vi "main.vi"() -> ()   [LabVIEW 2020]
uses:
  <vilib>/Math Plots/3D Math Plots/3D Scatter/3D Scatter XCtrl/3D Scatter.xctl
  <vilib>/Utility/miscctls.llb/LVRectTypeDef.ctl
  4961857f-4cb1-4452-8877-0132d1278599.vi
  3aed9957-f963-49bf-9f60-3d26462443e8.vi
  8fbe439c-06e5-460e-a560-e938ce784f44.vi
  460a15f0-0b3a-4794-87ef-3f3f720a4f09.vi
  13309ec4-5ddb-4caa-9ccb-149c6c5ba2b7.vi
  adf563d6-8bae-41a4-be26-81c21254c55c.vi
  <vilib>/Utility/inputDevices.llb/keyboardAcquire.vi
  <vilib>/Math Plots/3D Math Plots/3D Scatter/3D Scatter Datatype/Public/Plot Helper (Vector).vi
  <vilib>/Utility/inputDevices.llb/closeKeyboard.vi
  <vilib>/Math Plots/3D Math Plots/3D Scatter/3D Scatter Datatype/3D Scatter Datatype.lvclass
panel:
  in  "Motion Tab":enum32{"POSITION", "MEASUREMENT"}(tab)
  in  "Run Program":bool
  in  "Select Program":string(combo)="NONE"
  out "1st Key":T1(ring)
  in  "Next Button":bool
  in  "Previous Button":bool
  in  "Up Button":bool
  in  "Down Button":bool
  in  "Jog Axes":bool
  in  "Menu Ring":string(combo)
  in  "Move":bool
  in  "Axis 1 Distance":dbl format="%.2g"
  in  "Axis 0 Distance":dbl format="%.2g"
  in  "Axis 0 Speed":dbl format="%.2g"
  in  "Axis 1 Speed":dbl format="%.2g"
  in  "Axis 1 Acc":dbl format="%.2g"
  in  "Axis 0 Acc":dbl format="%.2g"
  in  "Set Parameters 2":bool
  in  "Axis 1 Jogspeed":dbl format="%.2g"
  in  "Axis 0 Jogspeed":dbl format="%.2g"
  in  "Track Offset\n(deg)":dbl format="%.2g"
  out "Data Points Logged":i32
  out "Laser Logging?":bool
  in  "Measurement\nAxis":i32(ring) items=["X Axis", "Y Axis"]
  in  "Travel Speed\n(mm/s)":dbl format="%.2g"
  in  "Set Parameters":bool
  in  "Ramp Distance\n(mm)":dbl min=0.0 format="%.2g"
  in  "Num Tracks":i32
  in  "Evaluation Length\n(mm)":dbl min=-90.0 max=90.0 format="%.2g"
  in  "Test Name":string
  out "Travel Dist":dbl
  in  "Travel Acc\n(mm/s2)":dbl format="%.2g"
  in  "Start Measurement":bool
  in  "Save Directory":path
  in  "STOP":bool
  in  "Setup Tab":enum32{"SETUP", "MONITORING", "ERRORS"}(tab)
  in  "Laser Offset":dbl
  in  "Home Axis":bool
  in  "Plot Laser Data":bool
  out "IsOpen":bool
  in  "Connection?":refnum<k7>(container)
  in  "Connect  to Controller":bool=TRUE
  in  "Set Parameters":bool
  in  "Controller Connection Type":string(combo)="2"
  out "Controller Type":string
  out "Product Name":string
  out "Version":string
  out "Serial Port":fxp<+,3,3>
  in  "Axis Enable":bool
  out "Lin Enc Pos":dbl format="%.3g"
  out "A Error":bool
  out "X Error":bool
  out "Axis 0 Position":dbl format="%.3f"
  out "Axis 0 End Pos":dbl format="%.3g"
  out "Axis 0 Velocity":dbl format="%.3g"
  out "A0 Remaining":dbl format="%.3g"
  out "XY Graph":cluster{"X":dbl, "Y":dbl}[](graph)
  out "A1 Remaining":dbl format="%.3g"
  out "Axis 1 End Pos":dbl format="%.3g"
  out "Axis 1 Velocity":dbl format="%.3g"
  out "Axis 1 Position":dbl format="%.3g"
  out "Rot Enc Pos":dbl format="%.3g"
  out "Loop Time (us)":u32
  out "Total Time Elapsed (s)":i32
  out "Controller  Error":errorcluster
  out "A Axis Error":errorcluster
  out "X Axis Error":errorcluster
  in  "Results Tab":enum32{"RESULTS"}(tab)
  out "Laser Displacement":dbl(graph)
  out "3D Plot":refnum<class "3D Plot Datatype.lvclass">[](xcontrol)
  # "DIRECT MOTION"
  # "SET PARAMETERS"
  # "SPEED \n(mm/s)"
  # "ACC / DEC\n(mm/s2)"
  # "JOGSPEED \n(mm/s)"
  # "X AXIS"
  # "X AXIS"
  # "(mm)"
  # "SPEED \n(deg/s)"
  # "ACC / DEC\n(deg/s2)"
  # "JOGSPEED \n(deg/s)"
  # "A AXIS"
  # "(deg)"
  # "A AXIS"
  # "AXIS JOGGING"
  # "A AXIS"
  # "X AXIS"
  # "KEYBOARD"
  # "CONTROLLER PROGRAMS"
  # "MEASUREMENT PARAMETERS"
  # "LASER DISPLACEMENT"
  # "CONTROLLER SETTINGS"
  # "LASER DISPLACEMENT SETTINGS"
  # "LINEAR AXIS FEEDBACK"
  # "Current Position \n(mm)"
  # "End Position \n(mm)"
  # "Travel Remaining \n(mm)"
  # "Velocity \n(mm/s2)"
  # "X AXIS"
  # "Encoder"
  # "ROTARY AXIS FEEDBACK"
  # "Current Position \n(deg)"
  # "End Position \n(deg)"
  # "Travel Remaining \n(deg)"
  # "Velocity \n(deg/s2)"
  # "A AXIS"
  # "Encoder"
  # "CONTROLLER"
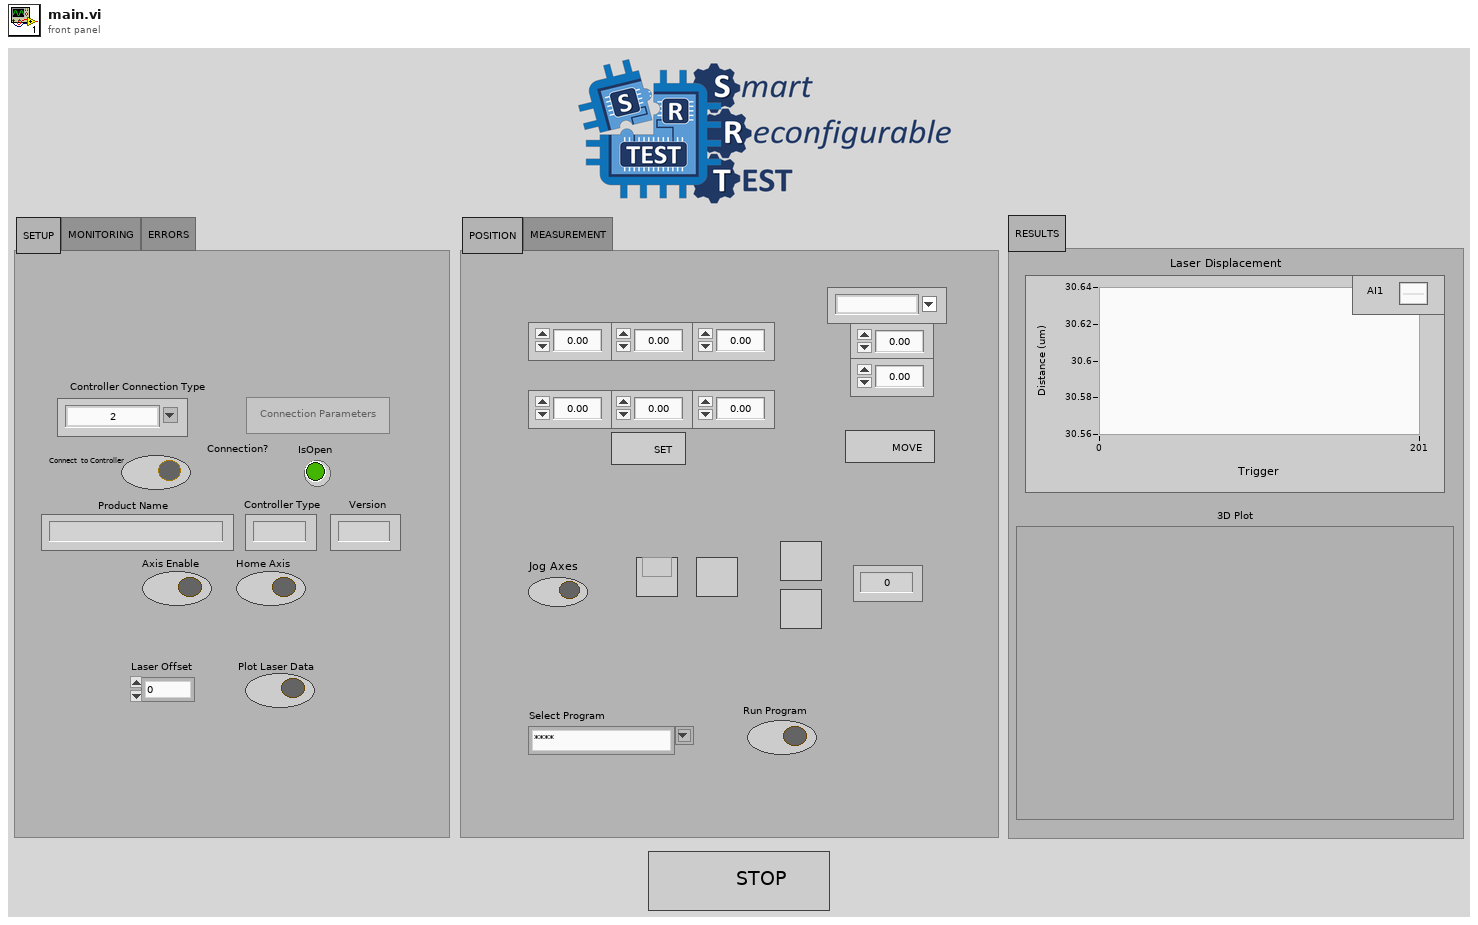
[diagram p1: front panel]
types:
  T1 = enum16{"0", "1", "2", "3", "4", "5", "6", "7", "8", "9", "A", "B", "C", "D", "E", "F", "G", "H", "I", "J", "K", "L", "M", "N", "O", "P", "Q", "R", "S", "T", "U", "V", "W", "X", "Y", "Z", "F1", "F2", "F3", "F4", "F5", "F6", "F7", "F8", "F9", "F10", "F11", "F12", "F13", "F14", "F15", "ADD", "BACK", "BACKSLASH", "CAPITAL", "COMMA", "DECIMAL", "DELETE", "DIVIDE", "DOWN", "END", "EQUALS", "ESCAPE", "GRAVE (`)", "HOME", "INSERT", "LBRACKET", "LCONTROL", "LEFT", "L ALT", "LSHIFT", "LWIN", "MINUS", "MULTIPLY", "NEXT", "NUMLOCK", "NUMPAD_0", "NUMPAD_1", "NUMPAD_2", "NUMPAD_3", "NUMPAD_4", "NUMPAD_5", "NUMPAD_6", "NUMPAD_7", "NUMPAD_8", "NUMPAD_9", "PAUSE", "PERIOD", "PRIOR (PG UP)", "RBRACKET", "RCONTROL", "RETURN", "RIGHT", "R ALT", "RSHIFT", "RWIN", "SCROLL", "SEMICOLON", "SLASH", "SPACE", "SUBTRACT", "TAB", "UP", "ENTER (num pad)", "' (quote)"}
  T2 = typedef "LVRectTypeDef.ctl" = cluster{"Left":i16, "Top":i16, "Right":i16, "Bottom":i16}
  T3 = enum8{"Enabled", "Disabled", "Disabled and Grayed Out"}
  T4 = enum16{"open", "replace", "create", "open or create", "replace or create", "replace or create with confirmation"}
  T5 = enum16{"0", "1", "2", "3", "4", "5", "6", "7", "8", "9", "A", "B", "C", "D", "E", "F", "G", "H", "I", "J", "K", "L", "M", "N", "O", "P", "Q", "R", "S", "T", "U", "V", "W", "X", "Y", "Z", "F1", "F2", "F3", "F4", "F5", "F6", "F7", "F8", "F9", "F10", "F11", "F12", "F13", "F14", "F15", "ADD", "BACK", "BACKSLASH", "CAPITAL", "COMMA", "DECIMAL", "DELETE", "DIVIDE", "DOWN", "END", "EQUALS", "ESCAPE", "GRAVE (`)", "HOME", "INSERT", "LBRACKET", "LCONTROL", "LEFT", "L ALT", "LSHIFT", "LWIN", "MINUS", "MULTIPLY", "NEXT", "NUMLOCK", "NUMPAD_0", "NUMPAD_1", "NUMPAD_2", "NUMPAD_3", "NUMPAD_4", "NUMPAD_5", "NUMPAD_6", "NUMPAD_7", "NUMPAD_8", "NUMPAD_9", "PAUSE", "PERIOD", "PRIOR (PG UP)", "RBRACKET", "RCONTROL", "RETURN", "RIGHT", "R ALT", "RSHIFT", "RWIN", "SCROLL", "SEMICOLON", "SLASH", "SPACE", "SUBTRACT", "TAB", "UP", "ENTER (num pad)", "' (quote)"}[]
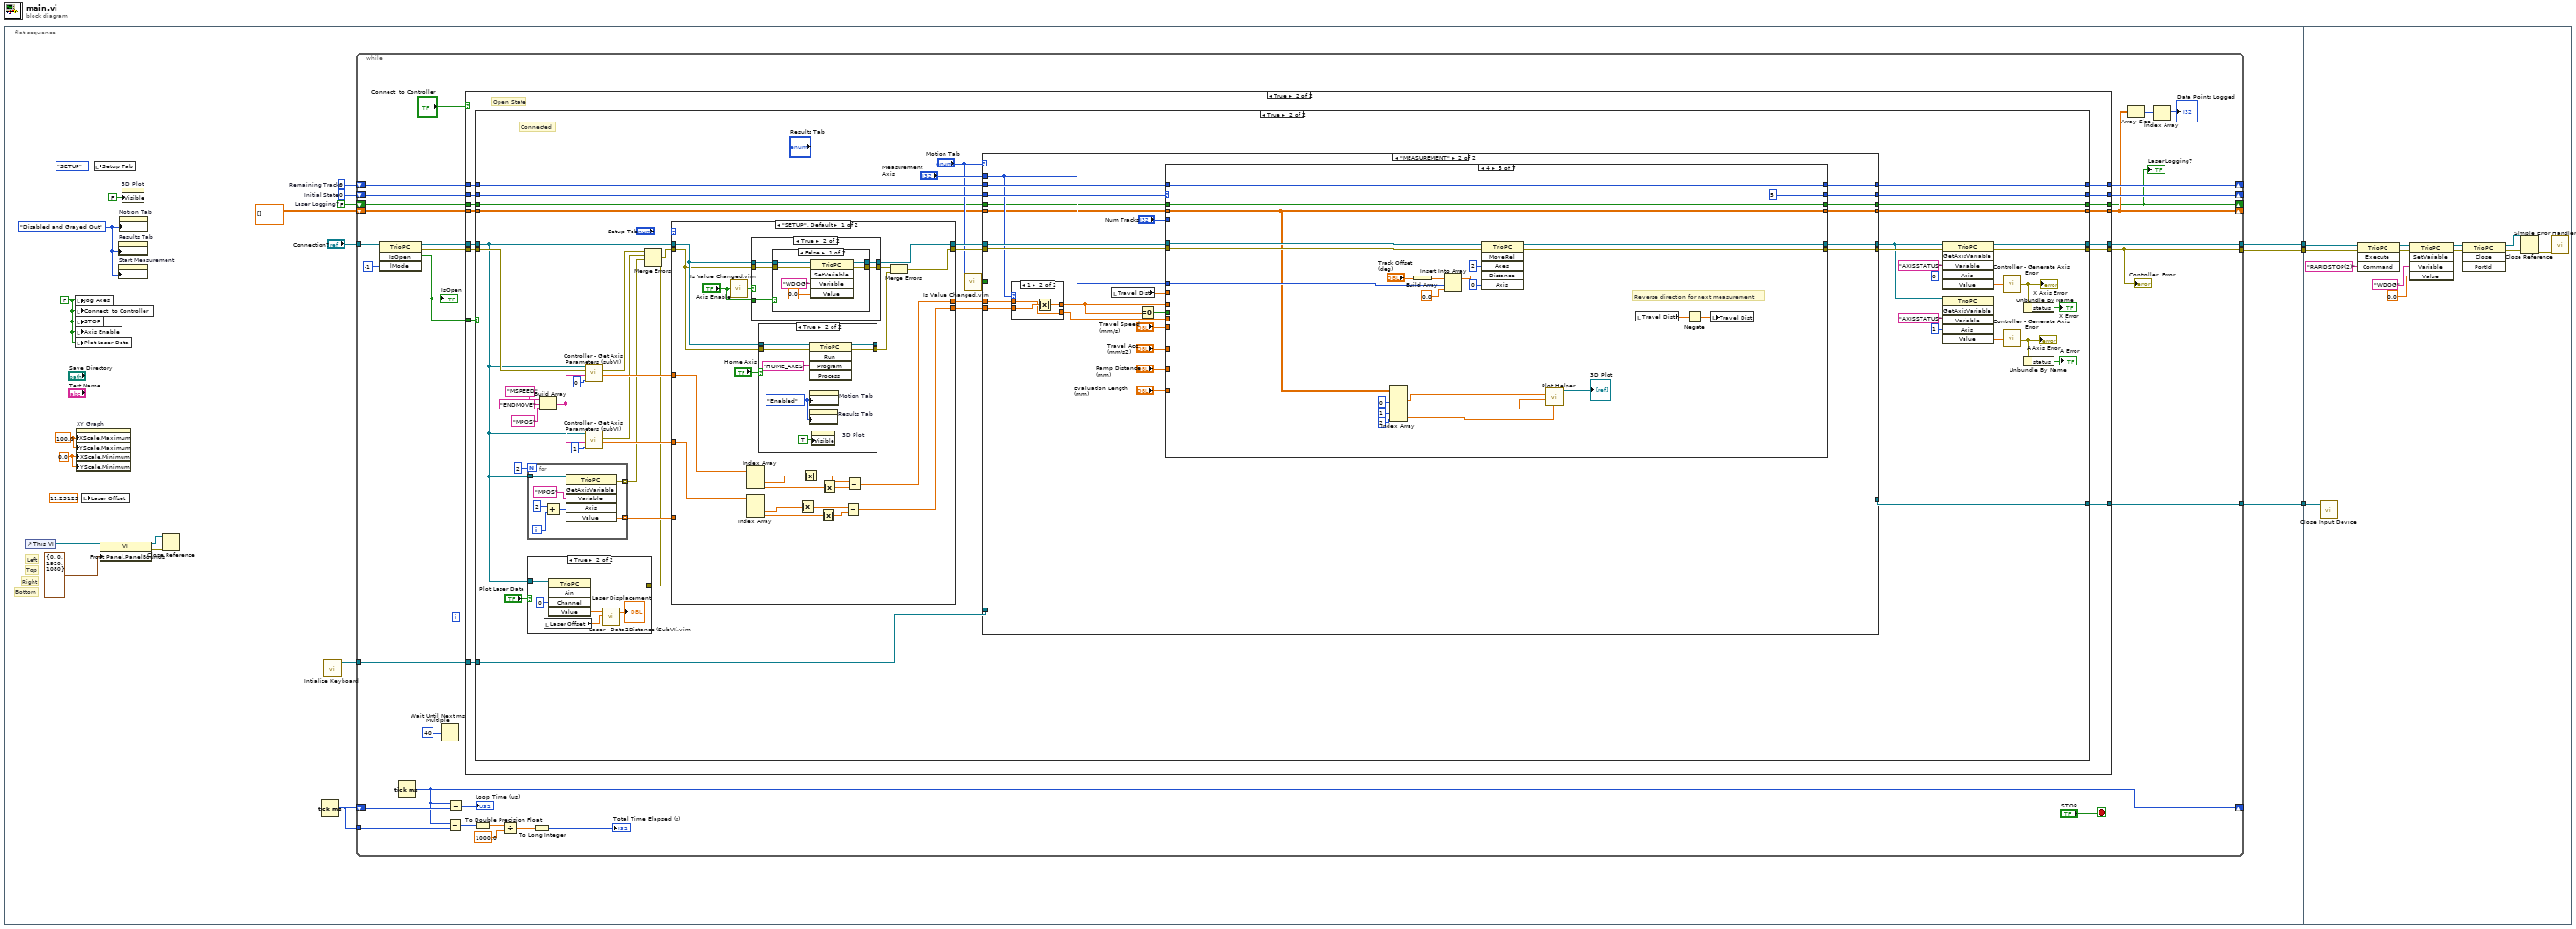
[diagram p0: block diagram]
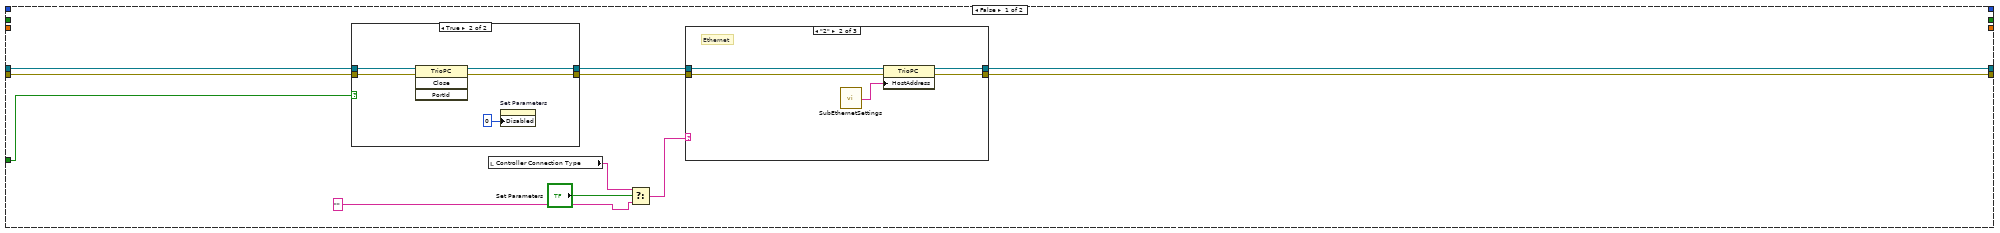
[diagram p2: hidden frame]
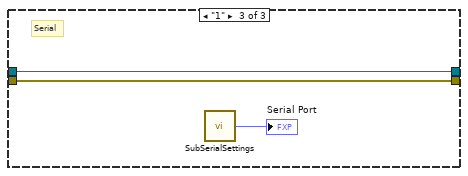
[diagram p5: hidden frame]
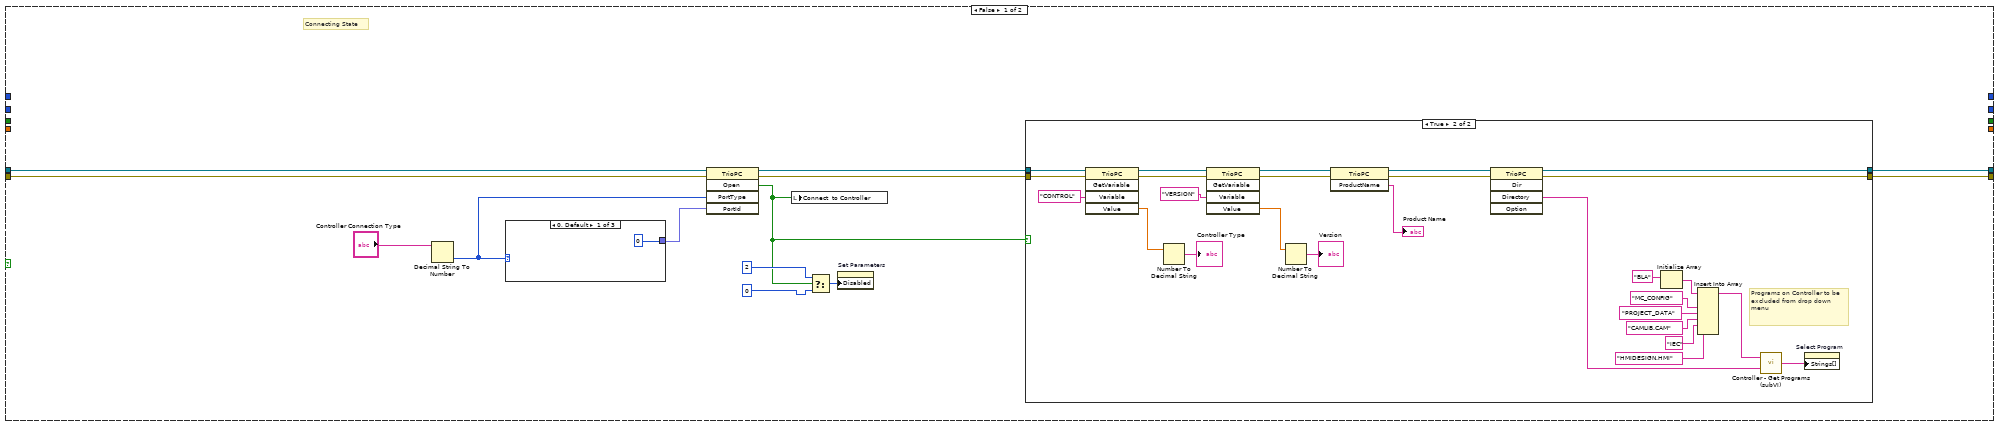
[diagram p6: hidden frame]
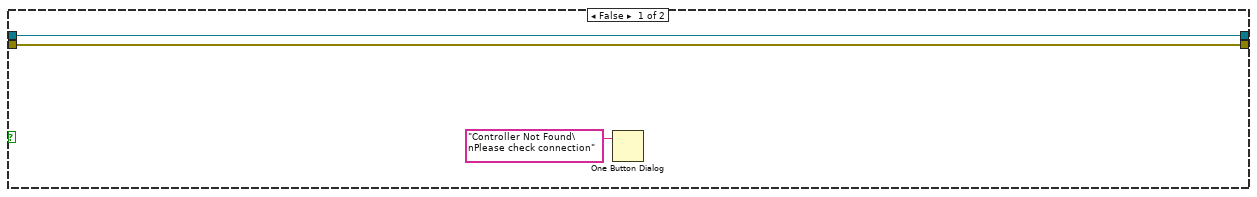
[diagram p7: hidden frame]
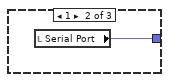
[diagram p8: hidden frame]
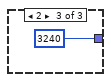
[diagram p9: hidden frame]
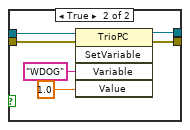
[diagram p13: hidden frame]
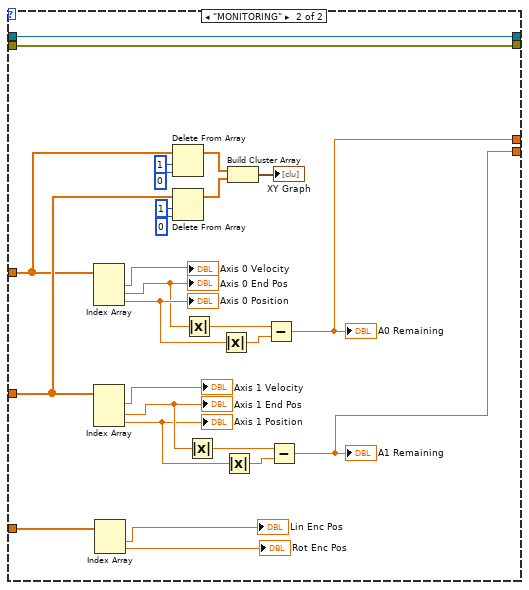
[diagram p14: hidden frame]
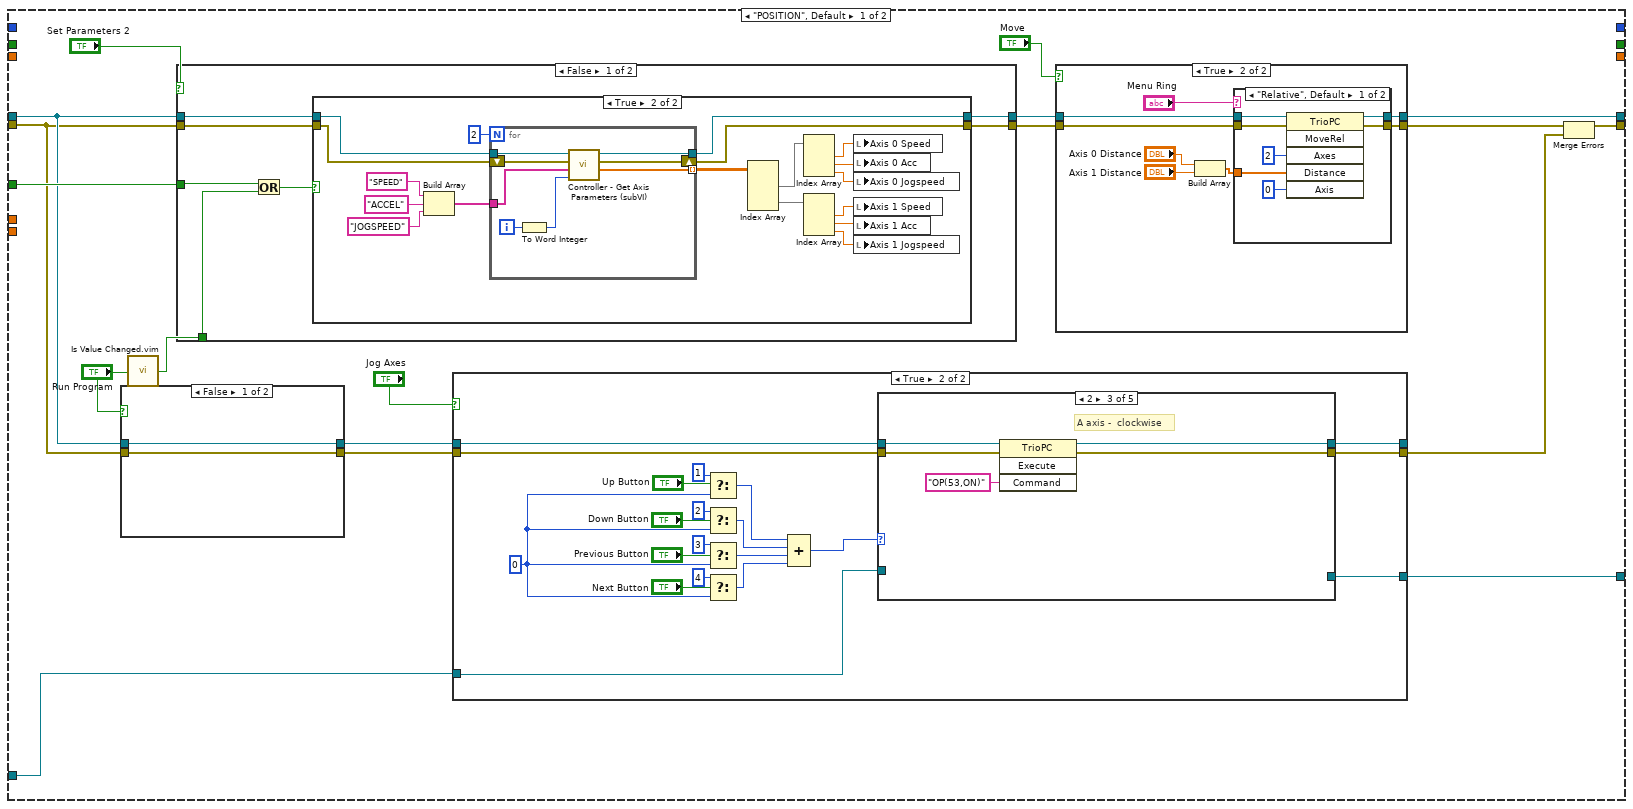
[diagram p15: hidden frame]
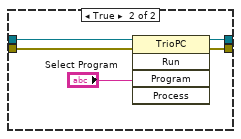
[diagram p16: hidden frame]
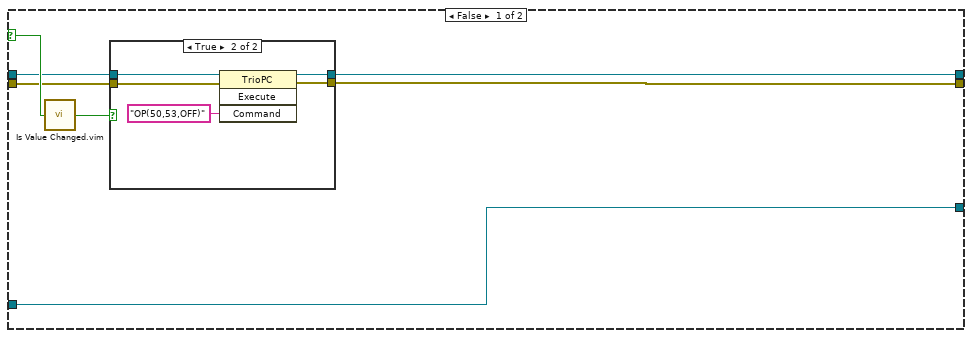
[diagram p17: hidden frame]
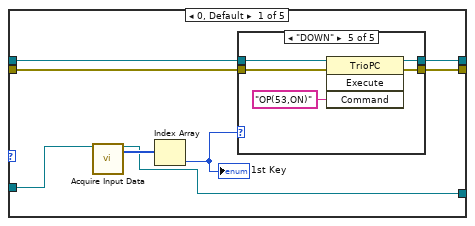
[diagram p19: hidden frame]
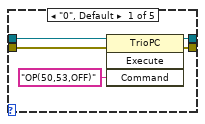
[diagram p20: hidden frame]
diagram:
  n1 = flat-sequence {
    tunnel: [w23] -> w3
    tunnel: [w22] -> w2
    tunnel: [w19] -> w1
    tunnel: w3 -> [w806]
    tunnel: w2 -> [w807]
    tunnel: w1 -> [w808]
    frame #0 {
      w5 = T3."Disabled and Grayed Out" ("Disabled")
      w14 = 0.0 ("X Scale.Range:Minimum")
      w13 = 100.0 ("X Scale.Range:Maximum")
      w12 = FALSE ("Jog Axes")
      # "Bottom"
      # "Right"
      # "Top"
      # "Left"
      n2 = control-ref of="This VI"() -> (w9:refnum<vi>)
      n3 = local write "Jog Axes"(w12) -> ()
      n4 = local write "Connect  to Controller"(w12) -> ()
      n5 = local write "STOP"(w12) -> ()
      n6 = local write "Axis Enable"(w12) -> ()
      n7 = local write "Plot Laser Data"(w12) -> ()
      n8 = property on="XY Graph" class="XYGraph (strict)"("XScale.Maximum"=w13, "YScale.Maximum"=w13, "XScale.Minimum"=w14, "YScale.Minimum"=w14) -> ()  [unwired: 2 in, 2 out]
      n9 = local write "Laser Offset"(11.23123 ("Laser Offset")) -> ()
      n10 = local write "Setup Tab"(enum32{"SETUP", "MONITORING", "ERRORS"}."SETUP" ("Setup Tab")) -> ()
      n11 = property class="VI"(reference=w9, "Front Panel.PanelBounds"=T2 {"Left"=0, "Top"=0, "Right"=1920, "Bottom"=1080} ("Front Panel Window:Panel Bounds")) -> (reference out=w6:refnum<vi>, error out=w7:errorcluster)  [unwired: 1 in]
      n12 = property on="Results Tab" class="TabCtl (strict)"("DisabledEnum"=w5) -> ()  [unwired: 2 in, 2 out]
      n13 = property on="Start Measurement" class="Bool"("DisabledEnum"=w5) -> ()  [unwired: 2 in, 2 out]
      n14 = property on="Motion Tab" class="TabCtl (strict)"("DisabledEnum"=w5) -> ()  [unwired: 2 in, 2 out]
      n15 = property on="3D Plot" class="3D Scatter (strict)"("Visible"=FALSE) -> ()  [unwired: 2 in, 2 out]
      n16 = Close Reference(reference=w6, error in (no error)=w7) -> ()  [unwired: 1 out]
    }
    frame #1 {
      w16 = FALSE  # Laser Logging?
      w17 = 0  # Remaining Tracks
      w18 = 0  # Initial State
      n17 = Tick Count (ms)() -> (millisecond timer value=w21:u32)
      n18 = call <vilib>:"Intialize Keyboard.vi"() -> ("device ID"=w20:refnum<k1>)  [unwired: 1 in, 10 out]
      n19 = while {
        tunnel: "Connection?" -> [w54]
        tunnel: [w51] -> w23
        tunnel: [w41] -> w22
        shift-right: [w44] -> _
        shift-left: w21 -> [w47]
        tunnel: w21 -> [w43]
        tunnel: w20 -> [w40]
        tunnel: [w39] -> w19
        shift-right: [w36] -> _
        shift-left: w18 -> [w35]
        shift-right: [w33] -> _
        shift-left: w17 -> [w34]
        shift-right: [w26] -> _
        shift-left: w16 -> [w30]
        shift-right: [w27] -> _
        shift-left: dbl[][] [] ("appended array") -> [w29]
        stop <- "STOP" stop-if-true
        n20 = invoke class="TrioPC" method="IsOpen"(reference=w54, "lMode"=-1) -> (reference out=w38:refnum<k7>, error out=w37:errorcluster, "IsOpen"=w52:bool)  [unwired: 2 in, 1 out]
        "IsOpen" <- w52
        n21 = Tick Count (ms)() -> (millisecond timer value=w44:u32)
        n22 = Wait Until Next ms Multiple(millisecond multiple=u32 40) -> ()  [unwired: 1 out]
        n23 = Subtract(x=w44, y=w43) -> (x-y=w42:u32)
        n24 = Subtract(x=w44, y=w47) -> (x-y=→"Loop Time (us)":u32)
        n25 = case shown="True" "Connect  to Controller" {
          tunnel: [w60 w98] -> w51
          tunnel: [w61 w97] -> w41
          tunnel: w52 -> [w57 w96]
          tunnel: w38 -> [w59 w95]
          tunnel: w37 -> [w58 w94]
          tunnel: w40 -> [_ w93]
          tunnel: [_ w92] -> w39
          tunnel: [_ w91] -> w36
          tunnel: w35 -> [_ w90]
          tunnel: w34 -> [_ w89]
          tunnel: [_ w88] -> w33
          tunnel: w30 -> [_ w87]
          tunnel: [_ w86] -> w27
          tunnel: w29 -> [_ w85]
          tunnel: [_ w84] -> w26
          frame False {
            n26 = case shown="True" w57 {
              tunnel: [w68 w73] -> w63
              tunnel: [w67 w72] -> w62
              tunnel: w59 -> [w68 w70]
              tunnel: w58 -> [w67 w69]
              frame False {
              }
              frame True {
                n27 = invoke class="TrioPC" method="Close"(reference=w70, error in=w69) -> (reference out=w73:refnum<k7>, error out=w72:errorcluster)  [unwired: 2 in, 2 out]
                n28 = property on="Set Parameters" class="Bool"("Disabled"=u8 0) -> ()  [unwired: 2 in, 2 out]
              }
            }
            n29 = local read "Controller Connection Type"() -> (w56:string)
            n30 = Select(t=w56, s="Set Parameters", f="") -> (s? t:f=w64:string)
            n31 = case shown="\"2\"" w64 {
              tunnel: w63 -> [w75 w78 w83]
              tunnel: w62 -> [w74 w77 w82]
              tunnel: [w75 w80 w83] -> w60
              tunnel: [w74 w79 w82] -> w61
              frame "", Default {
              }
              frame "2" {
                # "Ethernet"
                n32 = call "SubEthernetSettings.vi"() -> ("Ethernet IP Address 2"=w76:string)
                n33 = property class="TrioPC"(reference=w78, error in=w77, "HostAddress"=w76) -> (reference out=w80:refnum<k7>, error out=w79:errorcluster)
              }
              frame "1" {
                # "Serial"
                n34 = call "SubSerialSettings.vi"() -> ("CommPort"=→"Serial Port":fxp<+,3,3>)
              }
            }
          }
          frame True {
            # "Open State"
            n35 = case shown="True" w96 {
              tunnel: [w102 w184] -> w98
              tunnel: [w103 w179] -> w97
              tunnel: w95 -> [w107 w149]
              tunnel: w94 -> [w106 w162]
              tunnel: w93 -> [_ w194]
              tunnel: [_ w193] -> w92
              tunnel: [_ w191] -> w91
              tunnel: w90 -> [_ w190]
              tunnel: w89 -> [_ w189]
              tunnel: [_ w188] -> w88
              tunnel: w87 -> [_ w148]
              tunnel: [_ w147] -> w86
              tunnel: w85 -> [_ w146]
              tunnel: [_ w145] -> w84
              frame False {
                # "Connecting State"
                n36 = Decimal String To Number(string="Controller Connection Type") -> (number=w104:i32)  [unwired: 2 in, 1 out]
                n37 = case shown="0, Default" w104 {
                  tunnel: [i16 0 ("PortId") w143 i16 3240 ("PortId")] -> w111
                  frame 0, Default {
                  }
                  frame 1 {
                    n38 = local read "Serial Port"() -> (w143:fxp<+,3,3>)
                  }
                  frame 2 {
                  }
                }
                n39 = invoke class="TrioPC" method="Open"(reference=w107, error in=w106, "PortType"=w104, "PortId"=w111) -> (reference out=w101:refnum<k7>, error out=w100:errorcluster, "Open"=w99:bool)  [unwired: 1 in, 2 out]
                n40 = local write "Connect  to Controller"(w99) -> ()
                n41 = Select(t=u8 2, s=w99, f=u8 0 ("Disabled")) -> (s? t:f=w108:u8)
                n42 = property on="Set Parameters" class="Bool"("Disabled"=w108) -> ()  [unwired: 2 in, 2 out]
                n43 = case shown="True" w99 {
                  tunnel: [w113 w115] -> w103
                  tunnel: [w114 w116] -> w102
                  tunnel: w101 -> [w114 w117]
                  tunnel: w100 -> [w113 w123]
                  frame False {
                    n44 = One Button Dialog(message="Controller Not Found\nPlease check connection") -> ()  [unwired: 1 in, 1 out]
                  }
                  frame True {
                    # "Programs on Controller to be excluded from drop down menu"
                    n45 = invoke class="TrioPC" method="GetVariable"(reference=w117, error in=w123, "Variable"="CONTROL") -> (reference out=w125:refnum<k7>, error out=w124:errorcluster, "Value"=w129:dbl)  [unwired: 2 in, 2 out]
                    n46 = Number To Decimal String(number=w129) -> (decimal integer string=→"Controller Type":string)  [unwired: 1 in]
                    n47 = invoke class="TrioPC" method="GetVariable"(reference=w125, error in=w124, "Variable"="VERSION") -> (reference out=w121:refnum<k7>, error out=w122:errorcluster, "Value"=w128:dbl)  [unwired: 2 in, 2 out]
                    n48 = Number To Decimal String(number=w128) -> (decimal integer string=→"Version":string)  [unwired: 1 in]
                    n49 = invoke class="TrioPC" method="ProductName"(reference=w121, error in=w122) -> (reference out=w120:refnum<k7>, error out=w119:errorcluster, "ProductName"=→"Product Name":string)  [unwired: 1 in]
                    n50 = invoke class="TrioPC" method="Dir"(reference=w120, error in=w119) -> (reference out=w116:refnum<k7>, error out=w115:errorcluster, "Directory"=w140:string)  [unwired: 3 in, 2 out]
                    n51 = Initialize Array("BLA" ("element")) -> (w139:string[])  [unwired: 1 in]
                    n52 = Insert Into Array(array=w139, new element #1="MC_CONFIG" ("element"), new element #2="PROJECT_DATA" ("element"), new element #3="CAMLIB.CAM" ("element"), new element #4="IEC" ("element"), new element #5="HMIDESIGN.HMI") -> (w132:string[])  [unwired: 1 in]
                    n53 = call "Controller - Get Programs (subVI).vi"("Controller Directory"=w140, "Exclusion List"=w132) -> ("Programs List"=w141:string[])
                    n54 = property on="Select Program" class="CmbBox"("Strings[]"=w141) -> ()  [unwired: 2 in, 2 out]
                  }
                }
              }
              frame True {
                # "Connected"
                n55 = for {
                  N: 2 -> [_]
                  tunnel: [w203] -> w153 mode=indexing
                  tunnel: w149 -> [w202]
                  tunnel: [w201] -> w151 mode=indexing
                  i -> [w206]
                  n56 = Add(x=2, y=w206) -> (x+y=w207:i32)
                  n57 = invoke class="TrioPC" method="GetAxisVariable"(reference=w202, "Variable"="MPOS", "Axis"=w207) -> (error out=w201:errorcluster, "Value"=w203:dbl)  [unwired: 3 in, 4 out]
                }
                n58 = case shown="True" "Plot Laser Data" {
                  tunnel: w149 -> [_ w199]
                  tunnel: [_ w198] -> w150
                  frame False {
                  }
                  frame True {
                    n59 = local read "Laser Offset"() -> (w195:dbl)
                    n60 = invoke class="TrioPC" method="Ain"(reference=w199, "Channel"=i16 0) -> (error out=w198:errorcluster, "Value"=w197:dbl)  [unwired: 3 in, 3 out]
                    n61 = call "Laser - Data2Distance (SubVI).vim"("Laser Offset"=w195, "Raw Data"=w197) -> ("Distance Values"=→"Laser Displacement":dbl)  [unwired: 9 in]
                  }
                }
                n62 = Build Array("MSPEED", "ENDMOVE", "MPOS") -> (w163:string[])
                n63 = call "Controller - Get Axis Parameters (subVI).vi"("Axis"=i16 0, "Axis Parameters"=w163, "error in (no error)"=w162, "Automation Refnum in"=w149) -> ("Axis Parameter Values"=w164:dbl[], "error out"=w161:errorcluster)  [unwired: 5 in, 1 out]
                n64 = call "Controller - Get Axis Parameters (subVI).vi"("Axis"=i16 1, "Axis Parameters"=w163, "Automation Refnum in"=w149) -> ("Axis Parameter Values"=w165:dbl[], "error out"=w160:errorcluster)  [unwired: 6 in, 1 out]
                n65 = Merge Errors(w161, w160, w151, w150) -> (w159:errorcluster)
                n66 = case shown="\"SETUP\", Default" "Setup Tab" {
                  tunnel: w149 -> [w225 w261]
                  tunnel: [w224 w261] -> w158
                  tunnel: [w221 w260] -> w178
                  tunnel: [w208 w264] -> w177
                  tunnel: [w209 w265] -> w172
                  tunnel: w165 -> [w210 w263]
                  tunnel: w164 -> [w211 w262]
                  tunnel: w159 -> [w220 w260]
                  tunnel: w153 -> [_ w259]
                  frame "SETUP", Default {
                    n67 = call "Is Value Changed.vim"("value"="Axis Enable") -> ("changed or first call?"=w227:bool)
                    n68 = Index Array(array=w211) -> (element #2=w216:dbl, element #3=w217:dbl)  [unwired: 3 in, 1 out]
                    n69 = Index Array(array=w210) -> (element #2=w219:dbl, element #3=w218:dbl)  [unwired: 3 in, 1 out]
                    n70 = case shown="True" w227 {
                      tunnel: [w239 w244] -> w223
                      tunnel: w220 -> [w239 w241]
                      tunnel: w225 -> [w238 w243]
                      tunnel: "Axis Enable" -> [_ w242]
                      tunnel: [w238 w240] -> w224
                      frame False {
                      }
                      frame True {
                        n71 = case shown="False" w242 {
                          tunnel: [w246 w252] -> w244
                          tunnel: w241 -> [w247 w253]
                          tunnel: w243 -> [w248 w254]
                          tunnel: [w245 w251] -> w240
                          frame False {
                            n72 = invoke class="TrioPC" method="SetVariable"(reference=w248, error in=w247, "Variable"="WDOG", "Value"=0.0) -> (reference out=w245:refnum<k7>, error out=w246:errorcluster)  [unwired: 1 in, 3 out]
                          }
                          frame True {
                            n73 = invoke class="TrioPC" method="SetVariable"(reference=w254, error in=w253, "Variable"="WDOG", "Value"=1.0) -> (reference out=w251:refnum<k7>, error out=w252:errorcluster)  [unwired: 1 in, 3 out]
                          }
                        }
                      }
                    }
                    n74 = case shown="True" "Home Axis" {
                      tunnel: w225 -> [w230 w236]
                      tunnel: w220 -> [w229 w235]
                      tunnel: [w230 w234] -> _
                      tunnel: [w229 w233] -> w222
                      frame False {
                      }
                      frame True {
                        w232 = T3."Enabled" ("Disabled")
                        n75 = invoke class="TrioPC" method="Run"(reference=w236, error in=w235, "Program"="HOME_AXES") -> (reference out=w234:refnum<k7>, error out=w233:errorcluster)  [unwired: 2 in, 3 out]
                        n76 = property on="Results Tab" class="TabCtl (strict)"("DisabledEnum"=w232) -> ()  [unwired: 2 in, 2 out]
                        n77 = property on="Motion Tab" class="TabCtl (strict)"("DisabledEnum"=w232) -> ()  [unwired: 2 in, 2 out]
                        n78 = property on="3D Plot" class="3D Scatter (strict)"("Visible"=TRUE) -> ()  [unwired: 2 in, 2 out]
                      }
                    }
                    n79 = Absolute Value(x=w219) -> (abs(x)=w214:dbl)
                    n80 = Absolute Value(x=w216) -> (abs(x)=w212:dbl)
                    n81 = Absolute Value(x=w218) -> (abs(x)=w215:dbl)
                    n82 = Absolute Value(x=w217) -> (abs(x)=w213:dbl)
                    n83 = Subtract(x=w214, y=w215) -> (x-y=w208:dbl)
                    n84 = Subtract(x=w212, y=w213) -> (x-y=w209:dbl)
                    n85 = Merge Errors(w223, w222) -> (w221:errorcluster)
                  }
                  frame "MONITORING" {
                    n86 = Index Array(array=w262) -> (element #1=→"Axis 0 Velocity":dbl, element #2=w278:dbl, element #3=w279:dbl)  [unwired: 3 in]
                    "Axis 0 Position" <- w279
                    "Axis 0 End Pos" <- w278
                    n87 = Index Array(array=w263) -> (element #1=→"Axis 1 Velocity":dbl, element #2=w282:dbl, element #3=w281:dbl)  [unwired: 3 in]
                    "Axis 1 Position" <- w281
                    "Axis 1 End Pos" <- w282
                    n88 = Index Array(array=w259) -> (element #1=→"Lin Enc Pos":dbl, element #2=→"Rot Enc Pos":dbl)  [unwired: 2 in]
                    n89 = Delete From Array(array=w262, length=1, index=0) -> (array with subset deleted=w271:dbl[])  [unwired: 1 out]
                    n90 = Delete From Array(array=w263, length=1, index=0) -> (array with subset deleted=w270:dbl[])  [unwired: 1 out]
                    n91 = Absolute Value(x=w278) -> (abs(x)=w273:dbl)
                    n92 = Absolute Value(x=w282) -> (abs(x)=w275:dbl)
                    n93 = Absolute Value(x=w279) -> (abs(x)=w274:dbl)
                    n94 = Absolute Value(x=w281) -> (abs(x)=w276:dbl)
                    n95 = Build Cluster Array(w271, w270) -> (→"XY Graph":cluster{dbl, dbl}[])
                    n96 = Subtract(x=w273, y=w274) -> (x-y=w265:dbl)
                    "A0 Remaining" <- w265
                    n97 = Subtract(x=w275, y=w276) -> (x-y=w264:dbl)
                    "A1 Remaining" <- w264
                  }
                }
                n98 = call "Is Value Changed.vim"("value"="Motion Tab") -> ("changed or first call?"=w155:bool)
                n99 = case shown="\"MEASUREMENT\"" "Motion Tab" {
                  tunnel: w178 -> [w287 w502]
                  tunnel: [w296 w499] -> w185
                  tunnel: w158 -> [w288 w503]
                  tunnel: [w293 w504] -> w157
                  tunnel: w194 -> [w292 _]
                  tunnel: [w297 _] -> w193
                  tunnel: "Measurement\nAxis" -> [_ w494]
                  tunnel: [_ w509] -> w191
                  tunnel: w190 -> [_ w508]
                  tunnel: w189 -> [_ w507]
                  tunnel: [_ w506] -> w188
                  tunnel: w172 -> [_ w501]
                  tunnel: w177 -> [_ w500]
                  tunnel: w155 -> [w290 _]
                  tunnel: w148 -> [_ w490]
                  tunnel: [_ w489] -> w147
                  tunnel: w146 -> [_ w488]
                  tunnel: [_ w486] -> w145
                  frame "POSITION", Default {
                    n100 = case shown="False" "Run Program" {
                      tunnel: w287 -> [w302 w307]
                      tunnel: [w302 w306] -> w285
                      tunnel: w288 -> [w301 w305]
                      tunnel: [w301 w304] -> w286
                      frame False {
                      }
                      frame True {
                        n101 = invoke class="TrioPC" method="Run"(reference=w305, error in=w307, "Program"="Select Program") -> (reference out=w304:refnum<k7>, error out=w306:errorcluster)  [unwired: 2 in, 3 out]
                      }
                    }
                    n102 = call "Is Value Changed.vim"("value"="Run Program") -> ("changed or first call?"=w283:bool)
                    n103 = case shown="False" "Set Parameters 2" {
                      tunnel: [w398 w436] -> w299
                      tunnel: w288 -> [w401 w432]
                      tunnel: w287 -> [w400 w431]
                      tunnel: [w399 w430] -> w300
                      tunnel: w290 -> [w397 _]
                      tunnel: w283 -> [w396 _]
                      frame False {
                        n104 = Or(x=w397, y=w396) -> (x .or. y?=w395:bool)
                        n105 = case shown="True" w395 {
                          tunnel: w401 -> [w403 w416]
                          tunnel: w400 -> [w402 w413]
                          tunnel: [w403 w415] -> w399
                          tunnel: [w402 w414] -> w398
                          frame False {
                          }
                          frame True {
                            n106 = Build Array("SPEED", "ACCEL", "JOGSPEED") -> (w417:string[])
                            n107 = for {
                              N: 2 -> [_]
                              tunnel: w417 -> [w429]
                              tunnel: w416 -> [w428]
                              tunnel: [w425] -> w412 mode=indexing
                              tunnel: [w424] -> w415
                              shift-right: [w423] -> w414
                              shift-left: w413 -> [w422]
                              i -> [w427]
                              n108 = To Word Integer(number=w427) -> (16bit integer=w426:i16)
                              n109 = call "Controller - Get Axis Parameters (subVI).vi"("Axis"=w426, "Axis Parameters"=w429, "error in (no error)"=w422, "Automation Refnum in"=w428) -> ("Axis Parameter Values"=w425:dbl[], "error out"=w423:errorcluster, "Automation Refnum out"=w424:refnum<k7>)  [unwired: 5 in]
                            }
                            n110 = Index Array(array=w412) -> (element #1=w411:dbl[], element #2=w410:dbl[])  [unwired: 4 in]
                            n111 = Index Array(array=w411) -> (element #1=w409:dbl, element #2=w408:dbl, element #3=w407:dbl)  [unwired: 3 in]
                            n112 = Index Array(array=w410) -> (element #1=w405:dbl, element #2=w406:dbl, element #3=w404:dbl)  [unwired: 3 in]
                            n113 = local write "Axis 0 Speed"(w409) -> ()
                            n114 = local write "Axis 0 Acc"(w408) -> ()
                            n115 = local write "Axis 0 Jogspeed"(w407) -> ()
                            n116 = local write "Axis 1 Speed"(w405) -> ()
                            n117 = local write "Axis 1 Acc"(w406) -> ()
                            n118 = local write "Axis 1 Jogspeed"(w404) -> ()
                          }
                        }
                      }
                      frame True {
                        n119 = Build Array("Axis 0 Speed", "Axis 1 Speed") -> (w441:dbl[])
                        n120 = Build Array("Axis 0 Acc", "Axis 1 Acc") -> (w440:dbl[])
                        n121 = Build Array("Axis 0 Jogspeed", "Axis 1 Jogspeed") -> (w433:dbl[])
                        n122 = for {
                          N: 3 -> [_]
                          tunnel: w441 -> [w452] mode=indexing
                          tunnel: w440 -> [w451] mode=indexing
                          tunnel: w433 -> [w453] mode=indexing
                          shift-right: [w444] -> w436
                          shift-left: w431 -> [w448]
                          shift-right: [w445] -> w430
                          shift-left: w432 -> [w449]
                          i -> [w450]
                          n123 = invoke class="TrioPC" method="SetAxisVariable"(reference=w449, error in=w448, "Variable"="SPEED", "Axis"=w450, "Value"=w452) -> (reference out=w460:refnum<k7>, error out=w459:errorcluster)  [unwired: 1 in, 4 out]
                          n124 = invoke class="TrioPC" method="SetAxisVariable"(reference=w460, error in=w459, "Variable"="ACCEL", "Axis"=w450, "Value"=w451) -> (reference out=w458:refnum<k7>, error out=w457:errorcluster)  [unwired: 1 in, 4 out]
                          n125 = invoke class="TrioPC" method="SetAxisVariable"(reference=w458, error in=w457, "Variable"="DECEL", "Axis"=w450, "Value"=w451) -> (reference out=w447:refnum<k7>, error out=w446:errorcluster)  [unwired: 1 in, 4 out]
                          n126 = invoke class="TrioPC" method="SetAxisVariable"(reference=w447, error in=w446, "Variable"="JOGSPEED", "Axis"=w450, "Value"=w453) -> (reference out=w445:refnum<k7>, error out=w444:errorcluster)  [unwired: 1 in, 4 out]
                        }
                      }
                    }
                    n127 = case shown="True" "Jog Axes" {
                      selector: "Jog Axes" -> [w313 _]
                      tunnel: w292 -> [w314 w325]
                      tunnel: [w314 w324] -> w297
                      tunnel: w286 -> [w311 w327]
                      tunnel: w285 -> [w310 w326]
                      tunnel: [w309 w322] -> w289
                      tunnel: [w308 w323] -> _
                      frame False {
                        n128 = call "Is Value Changed.vim"("value"=w313) -> ("changed or first call?"=w312:bool)
                        n129 = case shown="True" w312 {
                          tunnel: [w316 w320] -> w308
                          tunnel: [w315 w319] -> w309
                          tunnel: w311 -> [w316 w318]
                          tunnel: w310 -> [w315 w317]
                          frame False {
                          }
                          frame True {
                            n130 = invoke class="TrioPC" method="Execute"(reference=w318, error in=w317, "Command"="OP(50,53,OFF)") -> (reference out=w320:refnum<k7>, error out=w319:errorcluster)  [unwired: 1 in, 2 out]
                          }
                        }
                      }
                      frame True {
                        w332 = 0 ("f")
                        n131 = Select(t=1, s="Up Button", f=w332) -> (s? t:f=w337:i32)
                        n132 = Select(t=2, s="Down Button", f=w332) -> (s? t:f=w336:i32)
                        n133 = Select(t=3, s="Previous Button", f=w332) -> (s? t:f=w335:i32)
                        n134 = Select(t=4, s="Next Button", f=w332) -> (s? t:f=w334:i32)
                        n135 = Compound Arithmetic op=ADD(w337, w336, w335, w334) -> (w333:i32)
                        n136 = case shown="2" w333 {
                          tunnel: w327 -> [w347 w378 w384 w388 w394]
                          tunnel: w326 -> [w346 w377 w383 w389 w393]
                          tunnel: [w345 w375 w382 w387 w392] -> w323
                          tunnel: [w344 w376 w381 w386 w391] -> w322
                          tunnel: w325 -> [w343 _ _ _ _]
                          tunnel: [w342 _ _ _ _] -> w324
                          frame 0, Default {
                            n137 = call-poly <vilib>:"Acquire Input Data.vi"("device ID"=w343) -> ("device ID"=w342:refnum<k1>, "keys pressed"=w348:T5)  [unwired: 1 in, 16 out]
                            n138 = Index Array(array=w348) -> (element=w349:T1)  [unwired: 1 in]
                            "1st Key" <- w349
                            n139 = case shown="\"DOWN\"" w349 {
                              tunnel: w347 -> [w354 w358 w364 w368 w374]
                              tunnel: w346 -> [w353 w359 w363 w367 w373]
                              tunnel: [w352 w357 w362 w365 w372] -> w345
                              tunnel: [w351 w356 w361 w366 w371] -> w344
                              frame "0", Default {
                                n140 = invoke class="TrioPC" method="Execute"(reference=w354, error in=w353, "Command"="OP(50,53,OFF)") -> (reference out=w352:refnum<k7>, error out=w351:errorcluster)  [unwired: 1 in, 2 out]
                              }
                              frame "LEFT" {
                                n141 = invoke class="TrioPC" method="Execute"(reference=w358, error in=w359, "Command"="OP(50,ON)") -> (reference out=w357:refnum<k7>, error out=w356:errorcluster)  [unwired: 1 in, 2 out]
                              }
                              frame "RIGHT" {
                                n142 = invoke class="TrioPC" method="Execute"(reference=w364, error in=w363, "Command"="OP(51,ON)") -> (reference out=w362:refnum<k7>, error out=w361:errorcluster)  [unwired: 1 in, 2 out]
                              }
                              frame "UP" {
                                n143 = invoke class="TrioPC" method="Execute"(reference=w368, error in=w367, "Command"="OP(52,ON)") -> (reference out=w365:refnum<k7>, error out=w366:errorcluster)  [unwired: 1 in, 2 out]
                              }
                              frame "DOWN" {
                                n144 = invoke class="TrioPC" method="Execute"(reference=w374, error in=w373, "Command"="OP(53,ON)") -> (reference out=w372:refnum<k7>, error out=w371:errorcluster)  [unwired: 1 in, 2 out]
                              }
                            }
                          }
                          frame 1 {
                            # "A axis anti-clockwise"
                            n145 = invoke class="TrioPC" method="Execute"(reference=w378, error in=w377, "Command"="OP(52,ON)") -> (reference out=w375:refnum<k7>, error out=w376:errorcluster)  [unwired: 1 in, 2 out]
                          }
                          frame 2 {
                            # "A axis -  clockwise"
                            n146 = invoke class="TrioPC" method="Execute"(reference=w384, error in=w383, "Command"="OP(53,ON)") -> (reference out=w382:refnum<k7>, error out=w381:errorcluster)  [unwired: 1 in, 2 out]
                          }
                          frame 3 {
                            # "X axis - left"
                            n147 = invoke class="TrioPC" method="Execute"(reference=w388, error in=w389, "Command"="OP(50,ON)") -> (reference out=w387:refnum<k7>, error out=w386:errorcluster)  [unwired: 1 in, 2 out]
                          }
                          frame 4 {
                            # "X axis - right"
                            n148 = invoke class="TrioPC" method="Execute"(reference=w394, error in=w393, "Command"="OP(51,ON)") -> (reference out=w392:refnum<k7>, error out=w391:errorcluster)  [unwired: 1 in, 2 out]
                          }
                        }
                      }
                    }
                    n149 = case shown="True" "Move" {
                      tunnel: [w463 w465] -> w293
                      tunnel: [w462 w464] -> w294
                      tunnel: w300 -> [w463 w468]
                      tunnel: w299 -> [w462 w467]
                      frame False {
                      }
                      frame True {
                        n150 = Build Array("Axis 0 Distance", "Axis 1 Distance") -> (w466:dbl[])
                        n151 = case shown="\"Relative\", Default" "Menu Ring" {
                          tunnel: w468 -> [w478 w484]
                          tunnel: w467 -> [w477 w483]
                          tunnel: w466 -> [w475 w480]
                          tunnel: [w473 w481] -> w465
                          tunnel: [w472 w482] -> w464
                          frame "Relative", Default {
                            n152 = invoke class="TrioPC" method="MoveRel"(reference=w478, error in=w477, "Axes"=i16 2, "Distance"=w475, "Axis"=0) -> (reference out=w473:refnum<k7>, error out=w472:errorcluster)  [unwired: 1 in, 4 out]
                          }
                          frame "Absolute" {
                            n153 = invoke class="TrioPC" method="MoveAbs"(reference=w484, error in=w483, "Axes"=i16 2, "Position"=w480, "Axis"=i16 0 ("Axes")) -> (reference out=w481:refnum<k7>, error out=w482:errorcluster)  [unwired: 1 in, 4 out]
                          }
                        }
                      }
                    }
                    n154 = Merge Errors(w294, w289) -> (w296:errorcluster)
                  }
                  frame "MEASUREMENT" {
                    n155 = case shown="1" w494 {
                      tunnel: w501 -> [w512 w513]
                      tunnel: w500 -> [w510 w515]
                      tunnel: [w511 w514] -> w492
                      tunnel: [w510 w513] -> w487
                      frame 0, Default {
                        n156 = Absolute Value(x=w512) -> (abs(x)=w511:dbl)
                      }
                      frame 1 {
                        n157 = Absolute Value(x=w515) -> (abs(x)=w514:dbl)
                      }
                    }
                    n158 = local read "Travel Dist"() -> (w505:dbl)
                    n159 = Equal To 0?(x=w492) -> (x = 0?=w493:bool)
                    n160 = case shown="4" w508 {
                      tunnel: w503 -> [w523 w586 w619 w697 w736 w744 w766]
                      tunnel: w502 -> [w522 w587 w620 w696 w735 w743 w758]
                      tunnel: w494 -> [_ w585 _ _ w727 _ _]
                      tunnel: [w525 w577 w617 w687 w733 w741 w757] -> w499
                      tunnel: [w524 w578 w618 w686 w734 w742 w766] -> w504
                      tunnel: [w530 w583 w615 4 ("Measurement\nAxis") 5 ("Measurement\nAxis") w745 w761] -> w509
                      tunnel: w507 -> [_ w582 w616 w711 w725 w747 w768]
                      tunnel: [w529 w582 w616 w711 w725 w746 w768] -> w506
                      tunnel: w493 -> [_ _ w624 _ _ _ _]
                      tunnel: w492 -> [_ _ w623 _ _ _ _]
                      tunnel: "Ramp Distance\n(mm)" -> [w521 w580 w622 _ _ _ _]
                      tunnel: w505 -> [_ w581 w621 _ _ _ _]
                      tunnel: "Travel Acc\n(mm/s2)" -> [w528 _ _ _ _ _ _]
                      tunnel: "Travel Speed\n(mm/s)" -> [w527 _ _ _ _ _ _]
                      tunnel: "Evaluation Length\n(mm)" -> [w526 _ _ _ _ _ _]
                      tunnel: "Num Tracks" -> [w519 _ _ _ _ _ _]
                      tunnel: w490 -> [w516 w576 w614 w685 w721 w737 w767]
                      tunnel: [w517 w575 w613 w694 w719 w738 dbl[][] [] ("appended array")] -> w489
                      tunnel: w488 -> [w517 w575 w613 w695 w719 w738 w759]
                      tunnel: w487 -> [_ _ _ _ _ w740 _]
                      tunnel: [w516 w574 w612 w685 w721 w737 w767] -> w486
                      frame 0, Default {
                        # "Not Measuring"
                        n161 = case shown="True" "Set Parameters" {
                          tunnel: [w537 w558] -> w524
                          tunnel: [w536 w557] -> w525
                          tunnel: w523 -> [w537 w544]
                          tunnel: w522 -> [w536 w542]
                          tunnel: w528 -> [_ w553]
                          tunnel: w527 -> [_ w552]
                          tunnel: w526 -> [_ w546]
                          tunnel: w521 -> [_ w551]
                          frame False {
                          }
                          frame True {
                            n162 = Absolute Value(x=w551) -> (abs(x)=w555:dbl)
                            n163 = Absolute Value(x=w546) -> (abs(x)=w550:dbl)
                            n164 = invoke class="TrioPC" method="Execute"(reference=w544, "Command"="NEW \"TABLE\"") -> (reference out=w540:refnum<k7>)  [unwired: 2 in, 3 out]
                            n165 = Multiply(x=w555, y=2.0) -> (x*y=w549:dbl)
                            n166 = Add(x=w549, y=w550) -> (x+y=w548:dbl)
                            n167 = Sign(1:w546) -> (0:w547:dbl)
                            n168 = Multiply(x=w548, y=w547) -> (x*y=→"Travel Dist":dbl)
                            n169 = invoke class="TrioPC" method="Execute"(reference=w540, error in=w542, "Command"="SCOPE(ON,20,0,3000,MPOS AXIS(2),MPOS AXIS(3),AIN(0))") -> (reference out=w543:refnum<k7>, error out=w541:errorcluster)  [unwired: 1 in, 2 out]
                            n170 = for {
                              N: 1 -> [_]
                              tunnel: w552 -> [w566]
                              tunnel: w553 -> [w565]
                              shift-right: [w560] -> w557
                              shift-left: w541 -> [w562]
                              shift-right: [w561] -> w558
                              shift-left: w543 -> [w563]
                              i -> [w564]
                              n171 = invoke class="TrioPC" method="SetAxisVariable"(reference=w563, error in=w562, "Variable"="SPEED", "Axis"=w564, "Value"=w566) -> (reference out=w572:refnum<k7>, error out=w571:errorcluster)  [unwired: 1 in, 4 out]
                              n172 = invoke class="TrioPC" method="SetAxisVariable"(reference=w572, error in=w571, "Variable"="ACCEL", "Axis"=w564, "Value"=w565) -> (reference out=w570:refnum<k7>, error out=w569:errorcluster)  [unwired: 1 in, 4 out]
                              n173 = invoke class="TrioPC" method="SetAxisVariable"(reference=w570, error in=w569, "Variable"="DECEL", "Axis"=w564, "Value"=w565) -> (reference out=w561:refnum<k7>, error out=w560:errorcluster)  [unwired: 1 in, 4 out]
                            }
                            n174 = property on="Start Measurement" class="Bool"("DisabledEnum"=T3."Enabled" ("Disabled")) -> ()  [unwired: 2 in, 2 out]
                          }
                        }
                        n175 = case shown="True" "Start Measurement" {
                          tunnel: [0 ("Axes") 1 ("Axes")] -> w530
                          tunnel: [0 ("f") w535] -> w529
                          tunnel: w519 -> [_ w535]
                          frame False {
                          }
                          frame True {
                            n176 = local write "Setup Tab"(enum32{"SETUP", "MONITORING", "ERRORS"}."MONITORING" ("Setup Tab")) -> ()
                          }
                        }
                      }
                      frame 1 {
                        # "Start Measurement Sequence"
                        n177 = Equal To 0?(x=w580) -> (x = 0?=w579:bool)
                        n178 = Not Equal To 0?(x=w582) -> (x != 0?=w584:bool)
                        n179 = case shown="True" w584 {
                          tunnel: w587 -> [w589 w603]
                          tunnel: w586 -> [w590 w602]
                          tunnel: w585 -> [_ w601]
                          tunnel: [w589 w592] -> w577
                          tunnel: [w590 w593] -> w578
                          tunnel: [6 ("Axes") 2 ("Axes")] -> w583
                          tunnel: w581 -> [_ w598]
                          tunnel: w579 -> [_ w597]
                          tunnel: [w588 w596] -> w574
                          tunnel: w576 -> [w588 _]
                          frame False {
                            # "Move to final state"
                            # "No Tracks to measure"
                          }
                          frame True {
                            n180 = invoke class="TrioPC" method="MoveRel"(reference=w602, error in=w603, "Axes"=i16 1, "Distance"=w598, "Axis"=w601) -> (reference out=w595:refnum<k7>, error out=w594:errorcluster)  [unwired: 1 in, 4 out]
                            n181 = case shown="True" w597 {
                              tunnel: [FALSE TRUE] -> w596
                              tunnel: w595 -> [w605 w610]
                              tunnel: w594 -> [w604 w609]
                              tunnel: [w605 w608] -> w593
                              tunnel: [w604 w607] -> w592
                              frame False {
                              }
                              frame True {
                                # "No Ramp Distance"
                                n182 = invoke class="TrioPC" method="Trigger"(reference=w610, error in=w609) -> (reference out=w608:refnum<k7>, error out=w607:errorcluster)  [unwired: 1 in, 1 out]
                              }
                            }
                          }
                        }
                      }
                      frame 2 {
                        # "Wait for Motion to Stop"
                        n183 = case shown="False" w624 {
                          tunnel: [2 ("Measurement\nAxis") 3 ("Measurement\nAxis")] -> w615
                          tunnel: w623 -> [w637 _]
                          tunnel: w622 -> [w636 _]
                          tunnel: w621 -> [w632 _]
                          tunnel: w620 -> [w628 w669]
                          tunnel: w619 -> [w630 w670]
                          tunnel: [w629 w670] -> w618
                          tunnel: [w627 w669] -> w617
                          tunnel: w614 -> [w626 _]
                          tunnel: [w625 FALSE] -> w612
                          frame False {
                            # "Axis Moving"
                            n184 = Absolute Value(x=w632) -> (abs(x)=w631:dbl)
                            n185 = Subtract(x=w631, y=w636) -> (x-y=w638:dbl)
                            n186 = Less Or Equal?(x=w637, y=w638) -> (x <= y?=w635:bool)
                            n187 = Greater Or Equal?(x=w637, y=w636) -> (x >= y?=w634:bool)
                            n188 = And(x=w635, y=w634) -> (x .and. y?=w633:bool)
                            n189 = case shown="False" w633 {
                              tunnel: w630 -> [w645 w660]
                              tunnel: [w642 w659] -> w629
                              tunnel: w628 -> [w644 w658]
                              tunnel: [w643 w657] -> w627
                              tunnel: w626 -> [w641 w656]
                              tunnel: [w640 w655] -> w625
                              frame False {
                                n190 = case shown="True" w641 {
                                selector: w641 -> [w646 _]
                                tunnel: w645 -> [w648 w654]
                                tunnel: w644 -> [w647 w653]
                                tunnel: [w647 w652] -> w643
                                tunnel: [w648 w650] -> w642
                                tunnel: [w646 FALSE] -> w640
                                frame False {
                                # "Axis Ramping Up"
                                }
                                frame True {
                                # "Axis Ramping Down"
                                n191 = invoke class="TrioPC" method="Execute"(reference=w654, error in=w653, "Command"="SCOPE(OFF)") -> (reference out=w650:refnum<k7>, error out=w652:errorcluster)  [unwired: 1 in, 2 out]
                                }
                                }
                              }
                              frame True {
                                # "Take Measurements"
                                n192 = case shown="False" w656 {
                                selector: w656 -> [_ w666]
                                tunnel: w660 -> [w665 w668]
                                tunnel: [w664 w668] -> w659
                                tunnel: w658 -> [w663 w667]
                                tunnel: [w662 w667] -> w657
                                tunnel: [TRUE w666] -> w655
                                frame False {
                                # "Start measurement"
                                n193 = invoke class="TrioPC" method="Trigger"(reference=w665, error in=w663) -> (reference out=w664:refnum<k7>, error out=w662:errorcluster)  [unwired: 1 in, 1 out]
                                }
                                frame True {
                                # "Measuring..."
                                }
                                }
                              }
                            }
                          }
                          frame True {
                            # "Track Movement Finished"
                          }
                        }
                      }
                      frame 3 {
                        w703 = 1000 ("index")
                        w708 = 3000 ("PortId")
                        # "Retreive stored data from controller and reset logging"
                        n194 = Initialize Array(0.0 ("disabled index (col)"), w708) -> (w706:dbl[])
                        n195 = invoke class="TrioPC" method="GetTable"(reference=w697, error in=w696, "StartPosition"=0 ("PortId"), "NumberOfValues"=w708, "Values"=w706) -> (reference out=w690:refnum<k7>, error out=w689:errorcluster, "Values"=w707:variant)  [unwired: 1 in, 3 out]
                        n196 = Variant To Data(type=w706, Variant=w707) -> (data=w705:dbl[])  [unwired: 1 in, 1 out]
                        n197 = Split 1D Array(array=w705, index=w703) -> (first subarray=w702:dbl[], second subarray=w704:dbl[])
                        n198 = Split 1D Array(array=w704, index=w703) -> (first subarray=w700:dbl[], second subarray=w698:dbl[])
                        n199 = Search 1D Array(1D array=w698, element=0.0) -> (index of element=w701:i32)  [unwired: 1 in]
                        n200 = Split 1D Array(array=w702, index=w701) -> (first subarray=w676:dbl[])  [unwired: 1 out]
                        n201 = Split 1D Array(array=w700, index=w701) -> (first subarray=w682:dbl[])  [unwired: 1 out]
                        n202 = Split 1D Array(array=w698, index=w701) -> (first subarray=w680:dbl[])  [unwired: 1 out]
                        n203 = expression code="(x/180.0)*pi" "deg2rad"(w682) -> (w681:dbl[])
                        n204 = call "Laser - Data2Distance (SubVI).vim"("Laser Offset"="Laser Offset", "Raw Data"=w680) -> ("Distance Values"=w677:dbl[])  [unwired: 9 in]
                        n205 = Sine & Cosine(0:w681) -> (1:w679:dbl[], 2:w678:dbl[])
                        n206 = Multiply(x=w679, y=w677) -> (x*y=w674:dbl[])
                        n207 = Multiply(x=w678, y=w677) -> (x*y=w673:dbl[])
                        n208 = Build Array(w676, w674, w673) -> (w684:dbl[][])
                        n209 = Transpose 2D Array(2D array=w684) -> (transposed array=w683:dbl[][])
                        n210 = Build Array (concatenate)(w695, w683) -> (w694:dbl[][])
                        n211 = invoke class="TrioPC" method="Execute"(reference=w690, error in=w689, "Command"="NEW \"TABLE\"") -> (reference out=w692:refnum<k7>, error out=w688:errorcluster)  [unwired: 1 in, 2 out]
                        n212 = invoke class="TrioPC" method="Execute"(reference=w692, error in=w688, "Command"="SCOPE(ON,20,0,3000,MPOS AXIS(2),MPOS AXIS(3),AIN(0))") -> (reference out=w686:refnum<k7>, error out=w687:errorcluster)  [unwired: 1 in, 2 out]
                      }
                      frame 4 {
                        # "Reverse direction for next measurement"
                        n213 = Index Array(array=w719, index (col) #1=0 ("disabled index (col)"), index (col) #2=1 ("index (col)"), index (col) #3=2 ("index (col)")) -> (element #1=w715:dbl[], element #2=w714:dbl[], element #3=w713:dbl[])  [unwired: 3 in]
                        n214 = Build Array("Track Offset\n(deg)") -> (w731:dbl[])
                        n215 = Insert Into Array(array=w731, index=w727, new element=0.0 ("new element/subarray")) -> (w730:dbl[])
                        n216 = invoke class="TrioPC" method="MoveRel"(reference=w736, error in=w735, "Axes"=i16 2, "Distance"=w730, "Axis"=i16 0 ("Axes")) -> (reference out=w734:refnum<k7>, error out=w733:errorcluster)  [unwired: 1 in, 4 out]
                        n217 = call-poly <vilib>:"Plot Helper.vi"("z vector"=w713, "y vector"=w714, "x vector"=w715) -> ("3D Plot lvclass Array out"=→"3D Plot":refnum<class "3D Plot Datatype.lvclass">[])  [unwired: 3 in, 5 out]
                        n218 = local read "Travel Dist"() -> (w724:dbl)
                        n219 = Negate(x=w724) -> (-x=w723:dbl)
                        n220 = local write "Travel Dist"(w723) -> ()
                      }
                      frame 5 {
                        # "Wait until offset complete and axis stopped"
                        n221 = Equal To 0?(x=w740) -> (x = 0?=w739:bool)
                        n222 = case shown="True" w739 {
                          tunnel: w747 -> [w751 w756]
                          tunnel: [w751 w755] -> w746
                          tunnel: [5 ("Measurement\nAxis") 1 ("Measurement\nAxis")] -> w745
                          tunnel: w744 -> [w749 w753]
                          tunnel: w743 -> [w748 w752]
                          tunnel: [w749 w753] -> w742
                          tunnel: [w748 w752] -> w741
                          frame False {
                            # "Still Moving"
                          }
                          frame True {
                            # "Start next measurement"
                            # "Finished Movement"
                            n223 = Decrement(x=w756) -> (x-1=w755:i32)
                          }
                        }
                      }
                      frame 6 {
                        n224 = Array Size(array=w759) -> (size(s)=w764:i32[])
                        n225 = Index Array(array=w764, index=0) -> (element=w763:i32)
                        n226 = Equal To 0?(x=w763) -> (x = 0?=w760:bool)
                        n227 = case shown="False" w760 {
                          tunnel: [0 ("Axes") 0 ("Axes")] -> w761
                          tunnel: w759 -> [w781 _]
                          tunnel: w758 -> [w774 w796]
                          tunnel: [w771 w796] -> w757
                          frame False {
                            n228 = local read "Save Directory"() -> (w792:path)
                            n229 = local read "Test Name"() -> (w795:string)
                            n230 = Path To String(path=w792) -> (string=w793:string)
                            n231 = Concatenate Strings(w793, "\\" ("string"), w795, ".csv" ("string")) -> (w794:string)
                            n232 = Array To Spreadsheet String(delimiter (Tab)=",", array=string[] ["Angle (deg)", "X Position (cm)", "Height (um)"], 3:"" ("format string")) -> (spreadsheet string=w783:string)
                            n233 = String To Path(string=w794) -> (path=w788:path)
                            n234 = Open/Create/Replace File(file path (use dialog)=w788, error in=w774, operation (0:open)=T4."replace or create with confirmation") -> (refnum out=w785:refnum<file>, error out=w786:errorcluster)  [unwired: 3 in, 1 out]
                            n235 = Write to Text File(file (use dialog)=w785, text=w783, error in=w786) -> (refnum out=w778:refnum<file>, error out=w777:errorcluster)  [unwired: 1 in, 1 out]
                            n236 = Array To Spreadsheet String(delimiter (Tab)=",", array=w781, 3:"%.6f" ("format string")) -> (spreadsheet string=w779:string)
                            n237 = Write to Text File(file (use dialog)=w778, text=w779, error in=w777) -> (refnum out=w775:refnum<file>, error out=w776:errorcluster)  [unwired: 1 in, 1 out]
                            n238 = Close File(refnum=w775, error in=w776) -> (error out=w772:errorcluster)  [unwired: 1 out]
                            n239 = call <vilib>:"Clear Errors.vi"("error in (no error)"=w772, "specific error code to clear (0: all)"=43) -> ("error out"=w771:errorcluster)  [unwired: 4 in, 1 out]
                          }
                          frame True {
                            # "No Data to Save"
                          }
                        }
                      }
                    }
                  }
                }
                n240 = invoke class="TrioPC" method="GetAxisVariable"(reference=w157, error in=w185, "Variable"="AXISSTATUS", "Axis"=i16 0) -> (reference out=w184:refnum<k7>, error out=w179:errorcluster, "Value"=w181:dbl)  [unwired: 2 in, 3 out]
                n241 = invoke class="TrioPC" method="GetAxisVariable"(reference=w157, "Variable"="AXISSTATUS", "Axis"=i16 1) -> ("Value"=w180:dbl)  [unwired: 3 in, 5 out]
                n242 = call "Controller - Generate Axis Error.vi"("Error Code"=w181) -> ("Error Description"=w174:errorcluster)
                "X Axis Error" <- w174
                n243 = call "Controller - Generate Axis Error.vi"("Error Code"=w180) -> ("Error Description"=w173:errorcluster)
                "A Axis Error" <- w173
                n244 = Unbundle By Name(w174) -> ("status"=→"X Error":bool)
                n245 = Unbundle By Name(w173) -> ("status"=→"A Error":bool)
              }
            }
          }
        }
        "Controller  Error" <- w41
        "Laser Logging?" <- w26
        n246 = To Double Precision Float(number=w42) -> (double precision float=w45:dbl)
        n247 = Divide(x=w45, y=1000.0) -> (x/y=w49:dbl)
        n248 = To Long Integer(number=w49) -> (32bit integer=→"Total Time Elapsed (s)":i32)
        n249 = Array Size(array=w27) -> (size(s)=w28:i32[])
        n250 = Index Array(array=w28) -> (element=→"Data Points Logged":i32)  [unwired: 1 in]
      }
    }
    frame #2 {
      n251 = call-poly <vilib>:"Close Input Device.vi"("device ID"=w808) -> ()  [unwired: 9 in, 1 out]
      n252 = invoke class="TrioPC" method="Execute"(reference=w806, error in=w807, "Command"="RAPIDSTOP(2)") -> (reference out=w802:refnum<k7>, error out=w803:errorcluster)  [unwired: 1 in, 2 out]
      n253 = invoke class="TrioPC" method="SetVariable"(reference=w802, error in=w803, "Variable"="WDOG", "Value"=0.0) -> (reference out=w801:refnum<k7>, error out=w800:errorcluster)  [unwired: 1 in, 3 out]
      n254 = invoke class="TrioPC" method="Close"(reference=w801, error in=w800) -> (reference out=w809:refnum<k7>, error out=w810:errorcluster)  [unwired: 2 in, 2 out]
      n255 = Close Reference(reference=w809, error in (no error)=w810) -> (error out=w805:errorcluster)
      n256 = call <vilib>:"Simple Error Handler.vi"("error in (no error)"=w805) -> ()  [unwired: 4 in, 5 out]
    }
  }
